vi "Numeric Indicator - Pendulum_2-08420.vi"() -> ()   [LabVIEW 2014]
panel:
  out "Pendulum":dbl(knob) scale=-5.0..5.0
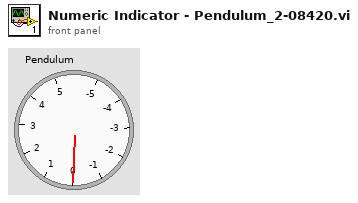
[diagram p1: front panel]
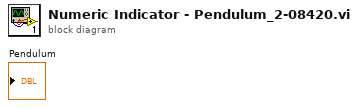
[diagram p0: block diagram]
diagram:
